vi "声参数计算.vi"(5 "错误输入":errorcluster caption="错误常量", 7 "Y":dbl[](array[numeric]), 8 "X":dbl[](array[numeric]), 10 "流道间隙":dbl) -> (0 "错误输出":errorcluster caption="错误常量", 3 "计算数据":dbl[](array[numeric]), 4 "声参数":dbl[](array[numeric]))   [LabVIEW 2018]
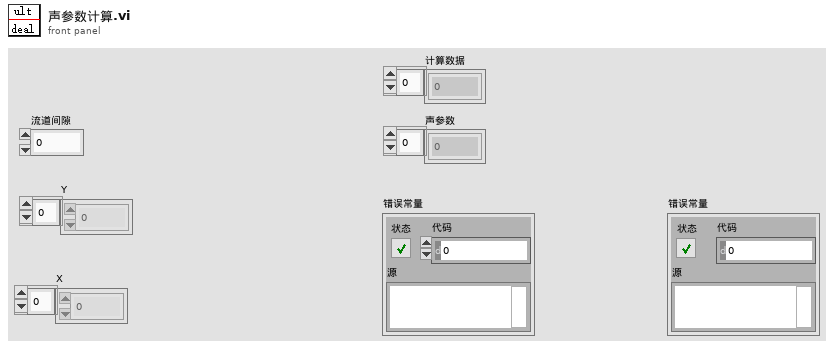
[diagram p1: front panel]
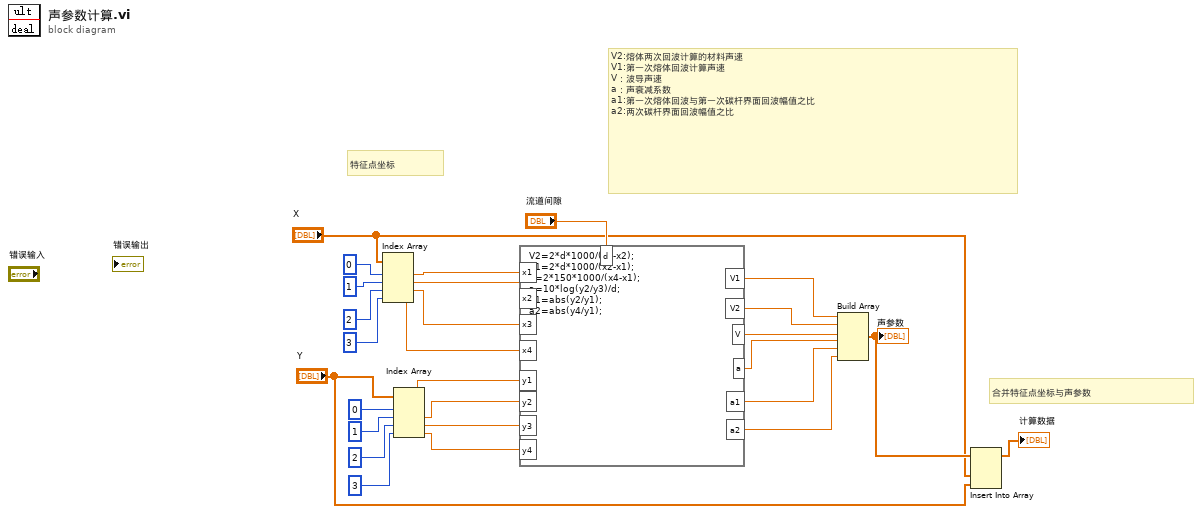
[diagram p0: block diagram]
diagram:
  # "合并特征点坐标与声参数"
  # "V2:熔体两次回波计算的材料声速\nV1:第一次熔体回波计算声速\nV：波导声速\na：声衰减系数\na1:第一次熔体回波与第一次碳杆界面回波幅值之比\na2:两次碳杆界面回波幅值之比"
  # "特征点坐标"
  n1 = Index Array(array="X", index #1=0 ("索引"), index #2=1 ("索引"), index #3=2 ("索引"), index #4=3 ("索引")) -> (element #1=w19:dbl, element #2=w18:dbl, element #3=w17:dbl, element #4=w16:dbl)
  n2 = Index Array(array="Y", index #1=0 ("索引"), index #2=1 ("索引"), index #3=2 ("索引"), index #4=3 ("索引")) -> (element #1=w15:dbl, element #2=w14:dbl, element #3=w13:dbl, element #4=w12:dbl)
  n3 = formula code="V2=2*d*1000/(x3-x2);\nV1=2*d*1000/(x2-x1);\nV=2*150*1000/(x4-x1);\na=10*log(y2/y3)/d;\na1=abs(y2/y1);\na2=abs(y4/y1);"("x1"=w19, "x2"=w18, "x3"=w17, "x4"=w16, "y2"=w14, "y3"=w13, "d"="流道间隙", "y1"=w15, "y4"=w12) -> ("V1"=w11:dbl, "V"=w9:dbl, "a"=w8:dbl, "a1"=w7:dbl, "a2"=w6:dbl, "V2"=w10:dbl)
  n4 = Build Array(w11, w10, w9, w8, w7, w6) -> (w4:dbl[])
  "声参数" <- w4
  n5 = Insert Into Array(array=w4, new element #1="X", new element #2="Y") -> (→"计算数据":dbl[])  [unwired: 1 in]
